vi "CONEX-ALL Get Last Command Error v2.vi"(11 "Connection Cluster in":T1) -> (1 "Error code":string, 3 "Connection Cluster out":T1)   [LabVIEW 2010]
doc: "TE? - Get Error\n\nQuery last Error code reported.\n\nReturn: Error code"
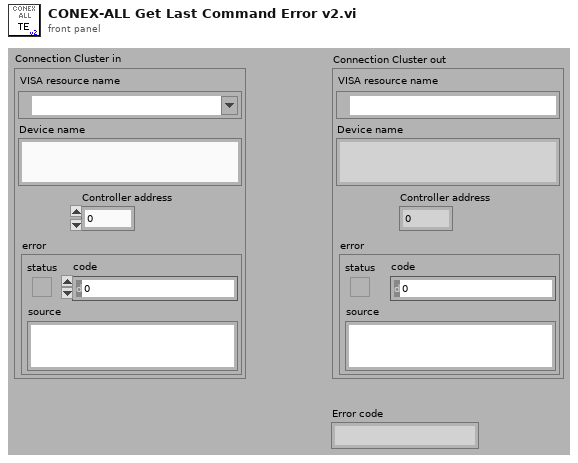
[diagram p1: front panel]
types:
  T1 = cluster{"VISA resource name":refnum<visa-resource-name>, "Device name":string, "Controller address":i32, "error":errorcluster}
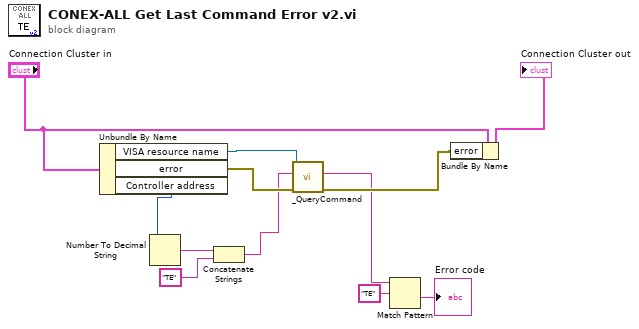
[diagram p0: block diagram]
diagram:
  n1 = Unbundle By Name("Connection Cluster in") -> ("VISA resource name"=w8:refnum<visa-resource-name>, "error"=w6:errorcluster, "Controller address"=w3:i32)
  n2 = Number To Decimal String(number=w3) -> (decimal integer string=w12:string)  [unwired: 1 out]
  n3 = Concatenate Strings(w12, "TE" ("strCommand")) -> (w2:string)
  n4 = call <userlib>:"_QueryCommand.vi"("error in"=w6, "Command"=w2, "Instrument Channel in"=w8) -> ("error out"=w7:errorcluster, "Response"=w1:string)  [unwired: 6 in, 1 out]
  n5 = Match Pattern(string=w1, regular expression="TE" ("expression régulière")) -> (after substring=→"Error code":string)  [unwired: 4 out]
  n6 = Bundle By Name(cluster="Connection Cluster in", "error"=w7) -> (→"Connection Cluster out":T1)
